vi "Data Dir.vi"(8 "error in (no error)":errorcluster, 11 "Name":string) -> (0 "error out":errorcluster, 2 "created":bool, 3 "path":path)   [LabVIEW 2014, in "lvprj2html.lvlib"]
uses:
  lvprj2html.lvlib
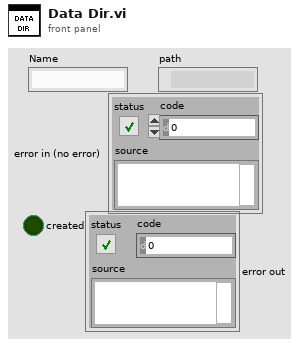
[diagram p1: front panel]
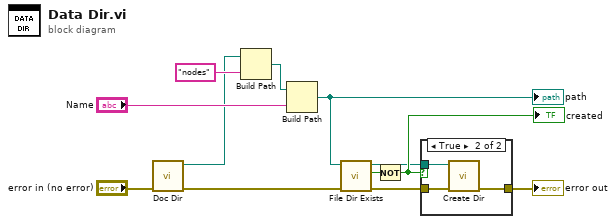
[diagram p0: block diagram]
diagram:
  n1 = call "Doc Dir.vi"("error in (no error)"="error in (no error)") -> ("error out"=w4:errorcluster, "appended path"=w10:path)  [unwired: 9 in]
  n2 = Build Path(base path=w10, name or relative path="nodes") -> (appended path=w9:path)
  n3 = Build Path(base path=w9, name or relative path="Name") -> (appended path=w5:path)
  "path" <- w5
  n4 = call "File Dir Exists.vi"("error in (no error)"=w4, "path"=w5) -> ("error out"=w1:errorcluster, "exists"=w3:bool, "path out"=w2:path)  [unwired: 7 in]
  n5 = Not(x=w3) -> (.not. x?=w6:bool)
  "created" <- w6
  n6 = case shown="True" w6 {
    tunnel: [w13 w16] -> w7
    tunnel: w2 -> [_ w15]
    tunnel: w1 -> [w13 w14]
    frame False {
    }
    frame True {
      n7 = call "Create Dir.vi"("error in (no error)"=w14, "appended path"=w15) -> ("error out"=w16:errorcluster)  [unwired: 8 in, 1 out]
    }
  }
  "error out" <- w7
